vi "Emballage_BDD_lecture_EMB_META.vi"(8 "Error in":errorcluster caption="Error in (no error)", 10 "CLE":string, 11 "ID_ARTICLE_GPAO":i32) -> (0 "Error out":errorcluster, 2 "Result Set":string[][](table) caption="Result Set (from first statement with results)", 3 "Column Names":string[](array[string]))   [LabVIEW 2020]
uses:
  Modules/FS/60_FS_Controles/60_FS_SetGet.ctl
  <vilib>/addons/database/Connection.llb/DB Tools Open Connec (Path).vi
  <vilib>/addons/database/Connection.llb/Conn Execute.vi
  <vilib>/addons/database/Recordset.llb/Rec Fetch Recordset Data (R).vi
  <vilib>/addons/database/Recordset.llb/Rec Destroy - Connection.vi
  <vilib>/addons/database/NI_Database_API.lvlib
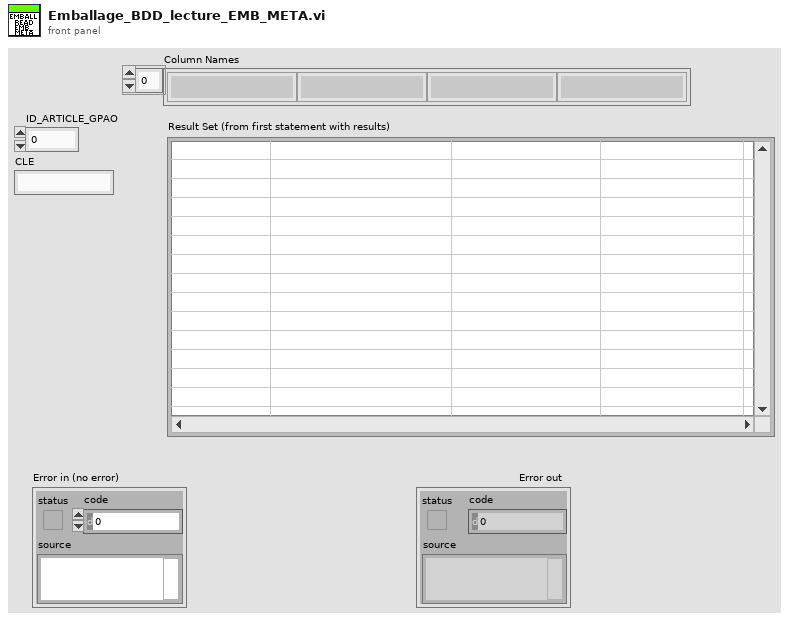
[diagram p1: front panel]
types:
  T1 = typedef "60_FS_SetGet.ctl" = enum16{"set", "get"}
  T2 = typedef "60_FS_CLT_Chemins.ctl" = cluster{"Racine_local":path, "Racine_reseau":path, "Racine_Support_Application":path, "Fichier_Journalisation":path, "Connexion_BDD_VSX":path, "Connexion_BDD_PLZ":path}
  T3 = typedef "NI_Database_API.lvlib/Conn ObjectReference.ctl" = refnum<k1>
  T4 = typedef "NI_Database_API.lvlib/Rec ObjectReference.ctl" = refnum<k1>
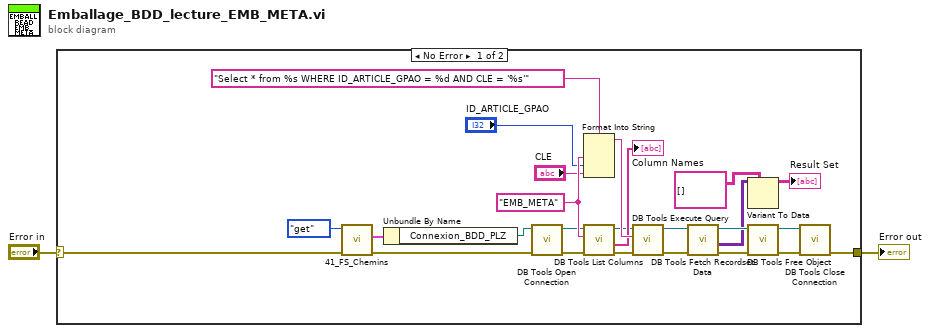
[diagram p0: block diagram]
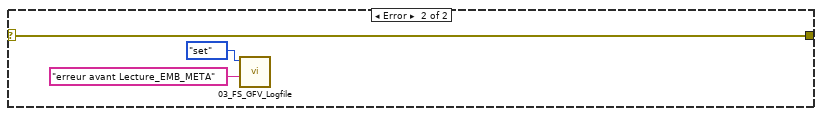
[diagram p2: hidden frame]
diagram:
  n1 = case shown="No Error" "Error in" {
    selector: "Error in" -> [w6 w30]
    tunnel: [w5 w30] -> w1
    frame No Error {
      w9 = "EMB_META" ("table")
      n2 = call "41_FS_Chemins.vi"("error in (no error)"=w6, "SetGet"=60_FS_SetGet."get") -> ("error out"=w17:errorcluster, "CLT_Chemins_out"=w25:T2)  [unwired: 8 in]
      n3 = Unbundle By Name(w25) -> ("Connexion_BDD_PLZ"=w18:path)
      n4 = call-poly <vilib>:"DB Tools Open Connection.vi"("error in (no error)"=w17, "connection information"=w18) -> ("error out"=w13:errorcluster, "connection reference"=w8:T3)  [unwired: 6 in]
      n5 = Format Into String(format string="Select * from %s WHERE ID_ARTICLE_GPAO = %d AND CLE = '%s'" ("SQL"), w9, "ID_ARTICLE_GPAO", "CLE") -> (resulting string=w16:string)  [unwired: 2 in, 1 out]
      n6 = call <vilib>:"DB Tools List Columns.vi"("error in (no error)"=w13, "table"=w9, "connection reference"=w8) -> ("error out"=w12:errorcluster, "columns"=→"Column Names":string[], "connection reference out"=w7:T3)  [unwired: 1 in, 1 out]
      n7 = call-poly <vilib>:"DB Tools Execute Query.vi"("error in (no error)"=w12, "SQL query"=w16, "connection reference"=w7) -> ("error out"=w22:errorcluster, "recordset reference"=w20:T4)  [unwired: 5 in]
      n8 = call-poly <vilib>:"DB Tools Fetch Recordset Data.vi"("error in (no error)"=w22, "recordset reference"=w20) -> ("error out"=w21:errorcluster, "recordset data"=w14:variant[][], "recordset reference out"=w19:T4)  [unwired: 3 in]
      n9 = Variant To Data(type=string[][] [] ("Liste des champs à lire 2"), Variant=w14) -> (data=→"Result Set":string[][])  [unwired: 1 in, 1 out]
      n10 = call-poly <vilib>:"DB Tools Free Object.vi"("error in (no error)"=w21, "recordset reference"=w19) -> ("error out"=w24:errorcluster, "connection reference"=w23:T3)  [unwired: 8 in]
      n11 = call <vilib>:"DB Tools Close Connection.vi"("error in (no error)"=w24, "connection reference"=w23) -> ("error out"=w5:errorcluster)  [unwired: 5 in]
    }
    frame Error {
      n12 = call "03_FS_GFV_Logfile.vi"("Chaîne"="erreur avant Lecture_EMB_META", "States"=60_FS_SetGet."set") -> ()  [unwired: 8 in, 2 out]
    }
  }
  "Error out" <- w1
